vi "XML Script - Append Terminal Name (For Loop Count).vi"(1 "for_loop":string) -> (0 "for_loop.Loop Count":string)   [LabVIEW 2017]
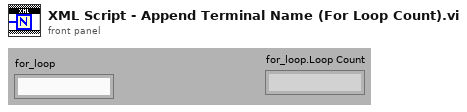
[diagram p1: front panel]
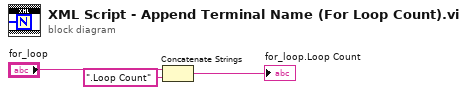
[diagram p0: block diagram]
diagram:
  n1 = Concatenate Strings("for_loop", ".Loop Count" ("string")) -> (→"for_loop.Loop Count":string)
